vi "Calculate Particle Scores.vi"(7 "Pixel Value":i32=1, 8 "Limit Tests?":bool, 9 "Aspect Fudge Factor":dbl=1.0, 10 "Sorted Data":dbl[][](array[numeric]), 11 "Image in":T2) -> (3 "Scores":T1(array[cluster]))   [LabVIEW 2014]
doc: "Calculate scores based on the particle measurements. Example scores are for trapezoidal area, aspect ratio, ratio of area to convex hull area, and masking for _| |_ shapes. These scores can later help to categorize particles into nonTargets, long targets, and short targets. The fudge factor compensates for camera modes that do not give square pixels."
uses:
  <vilib>/vision/Image Controls.llb/IMAQ Image.ctl
  <vilib>/vision/NI_Vision_Development_Module.lvlib
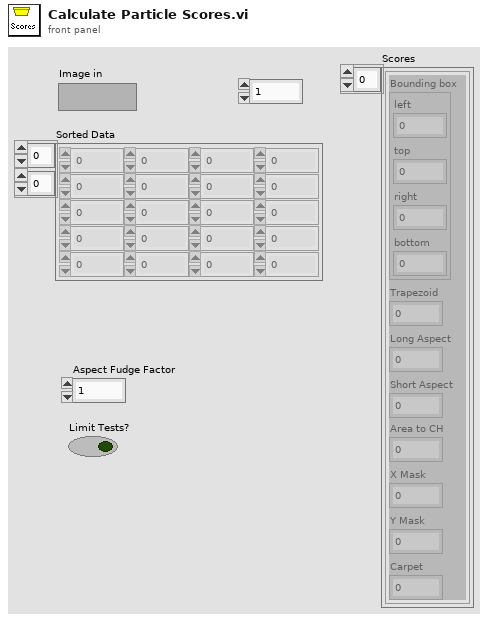
[diagram p1: front panel]
types:
  T1 = cluster{"Bounding box":cluster{"left":dbl, "top":dbl, "right":dbl, "bottom":dbl}, "Trapezoid":dbl, "Long Aspect":dbl, "Short Aspect":dbl, "Area to CH":dbl, "X Mask":dbl, "Y Mask":dbl, "Carpet":dbl}[]
  T2 = typedef "IMAQ Image.ctl" = refnum<image>
  T3 = cluster{"[0]":dbl, "[1]":dbl, "[2]":dbl, "[3]":dbl}
  T4 = cluster{cluster{"[0]":dbl, "[1]":dbl, "[2]":dbl, "[3]":dbl}, "Score":dbl, "Long Edge Score":dbl, "Short Edge Score":dbl, "Score":dbl, "X Score":dbl, "Y Score":dbl, "Carpet":dbl}
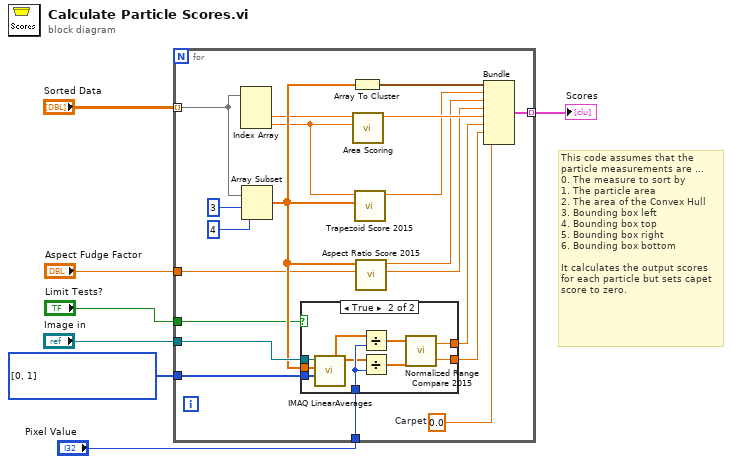
[diagram p0: block diagram]
diagram:
  w5 = i32[] [0, 1] items=["X Axis Averages", "Y Axis Averages", "X + Y Axis Averages", "X - Y Axis Averages"] ("Averages")
  # "This code assumes that the\nparticle measurements are ...\n0. The measure to sort by\n1. The particle area\n2. The area of the Convex Hull\n3. Bounding box left\n4. Bounding box top\n5. Bounding box right\n6. Bounding box bottom\n\nIt calculates the output scores\nfor each particle but sets capet\nscore to zero."
  n1 = for {
    tunnel: "Image in" -> [w22]
    tunnel: "Sorted Data" -> [w25] mode=indexing
    tunnel: [w24] -> w6 mode=indexing
    tunnel: w5 -> [w16]
    tunnel: "Pixel Value" -> [w12]
    tunnel: "Aspect Fudge Factor" -> [w9]
    tunnel: "Limit Tests?" -> [w8]
    w14 = 0.0  # Carpet
    n2 = Index Array(array=w25) -> (element #2=w11:dbl, element #3=w10:dbl)  [unwired: 3 in, 1 out]
    n3 = Array Subset(array=w25, index=3, length=4) -> (w13:dbl[])
    n4 = case shown="True" w8 {
      tunnel: w22 -> [_ w37]
      tunnel: [_ w36] -> w18
      tunnel: [_ w35] -> w17
      tunnel: w16 -> [_ w34]
      tunnel: w13 -> [_ w33]
      tunnel: w12 -> [_ w32]
      frame False {
      }
      frame True {
        n5 = call "IMAQ LinearAverages"("Averages"=w34, "Optional Rectangle"=w33, "Image Src"=w37) -> ("Y Axis Averages"=w30:sgl[], "X Axis Averages"=w31:sgl[])  [unwired: 4 in, 3 out]
        n6 = Divide(x=w31, y=w32) -> (x/y=w29:sgl[])
        n7 = Divide(x=w30, y=w32) -> (x/y=w28:sgl[])
        n8 = call "Normalized Range Compare 2015.vi"("Y Averages"=w28, "X Averages"=w29) -> ("Y Score"=w35:dbl, "X Score"=w36:dbl)
      }
    }
    n9 = Array To Cluster(array=w13) -> (cluster=w21:T3)
    n10 = call "Area Scoring.vi"("Convex Hull Area"=w10, "Area"=w11) -> ("Score"=w23:dbl)  [unwired: 9 in]
    n11 = call "Trapezoid Score 2015.vi"("Rectangle Array ltrb"=w13, "Convex Hull Area"=w10) -> ("Score"=w20:dbl)  [unwired: 9 in]
    n12 = call "Aspect Ratio Score 2015.vi"("Aspect Fudge Factor"=w9, "Rectangle Array ltrb"=w13) -> ("Short Edge Score"=w15:dbl, "Long Edge Score"=w19:dbl)  [unwired: 8 in]
    n13 = Bundle(w21, "Score"=w20, "Long Edge Score"=w19, "Short Edge Score"=w15, "Score"=w23, "X Score"=w18, "Y Score"=w17, "Carpet"=w14) -> (w24:T4)  [unwired: 1 in]
  }
  "Scores" <- w6
